vi "UE9 ms Multiple Pulse Output.vi"(8 "error in":errorcluster) -> ()   [LabVIEW 2021]
panel:
  in  "Number of Pulses":u16=1
  in  "Pulse Width (ms)":dbl=10.0 min=1.0 max=260.0 step=1.0
  in  "FirstFound":bool=TRUE
  in  "Address":string="1"
  out "Error Message":string
  # "Demonstrates using a PWM output and a stop timer to create multiple pulses with a pulse width\nfrom 1-260 ms which is variable in 1 ms increments.  Frequency of the pulses is 3.8 Hz.  The PWM\noutput is on FIO0, and the stop timer is on FIO1, so FIO0 must be shorted to FIO1 for the stop\ntimer to work.\n\nThe pulses are negative (signal is normally-high).  If positive pulses are needed, an inverter IC\nshould be put on the signal."
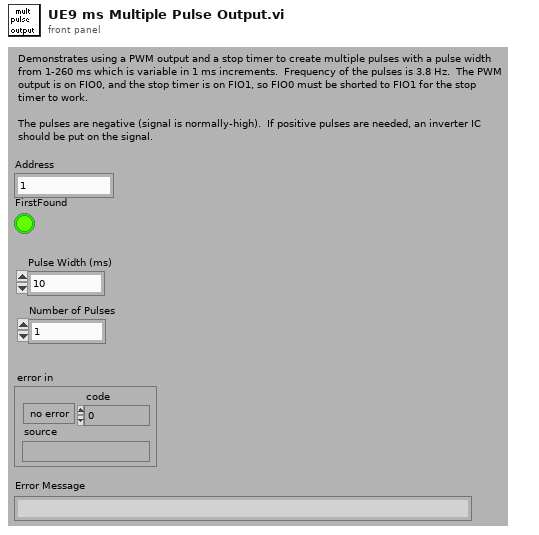
[diagram p1: front panel]
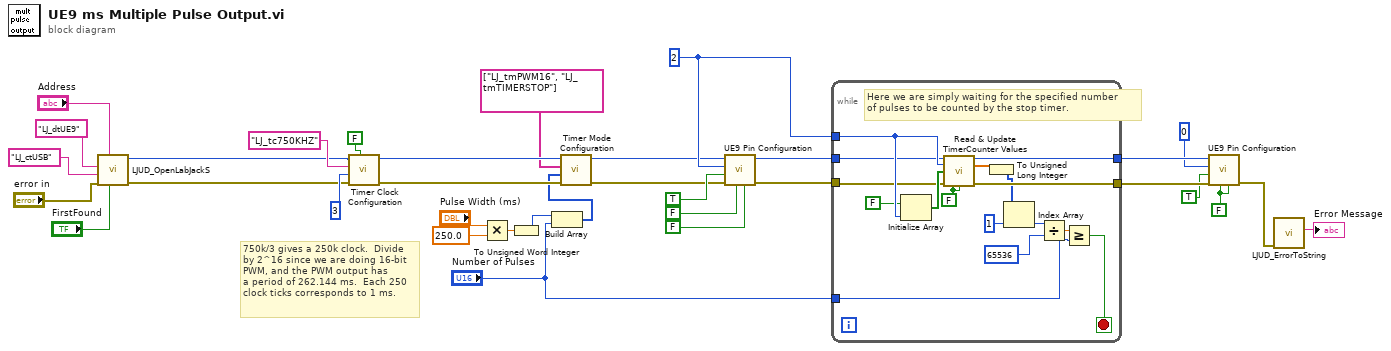
[diagram p0: block diagram]
diagram:
  w8 = FALSE ("Enable Counter0")
  w11 = u8 2 ("Number of Timers Enabled")
  # "750k/3 gives a 250k clock.  Divide\nby 2^16 since we are doing 16-bit\nPWM, and the PWM output has\na period of 262.144 ms.  Each 250\nclock ticks corresponds to 1 ms."
  n1 = call "LJUD_OpenLabJackS.vi"("FirstFound"="FirstFound", "Address"="Address", "error in"="error in", "ConnectionType"="LJ_ctUSB", "DeviceType"="LJ_dtUE9") -> ("error out"=w5:errorcluster, "Handle"=w6:i32)  [unwired: 4 in, 1 out]
  n2 = call "Timer Clock Configuration.vi"("Do Not Do Go()"=FALSE, "error in"=w5, "Timer Clock Divisor"=3, "Timer Clock Base"="LJ_tc750KHZ", "Handle In"=w6) -> ("error out"=w22:errorcluster, "Handle Out"=w21:i32)  [unwired: 5 in]
  n3 = Multiply(x="Pulse Width (ms)", y=250.0) -> (x*y=w15:dbl)
  n4 = To Unsigned Word Integer(number=w15) -> (unsigned 16bit integer=w12:u16)
  n5 = Build Array(w12, "Number of Pulses") -> (w14:u16[])
  n6 = call "Timer Mode Configuration.vi"("error in"=w22, "TimerValues"=w14, "TimerModes"=string[] ["LJ_tmPWM16", "LJ_tmTIMERSTOP"], "Handle In"=w21) -> ("error out"=w3:errorcluster, "Handle Out"=w4:i32)  [unwired: 6 in]
  n7 = call "UE9 Pin Configuration.vi"("Enable Counter1"=FALSE ("Enable Counter0"), "Enable Counter0"=FALSE, "error in"=w3, "Enable DACs"=TRUE ("Enable Counter0"), "Number of Timers Enabled"=w11, "Handle In"=w4) -> ("error out"=w2:errorcluster, "Handle Out"=w1:i32)  [unwired: 4 in]
  n8 = while {
    tunnel: [w50] -> w10
    tunnel: [w48] -> w30
    tunnel: w11 -> [w47]
    tunnel: w1 -> [w45]
    tunnel: w2 -> [w44]
    tunnel: "Number of Pulses" -> [w35]
    stop <- w37 stop-if-true
    w46 = FALSE ("Reset Counter0")
    # "Here we are simply waiting for the specified number\nof pulses to be counted by the stop timer."
    n9 = Initialize Array(FALSE, w47) -> (w49:bool[])
    n10 = call "Read & Update TimerCounter Values.vi"("Handle In"=w45, "# Timers to Read"=w47, "UpdateReset Timers"=w49, "error in"=w44, "Read Counter0"=w46, "Read Counter1"=w46) -> ("Handle Out"=w48:i32, "Timer Value Reads"=w39:dbl[], "error out"=w50:errorcluster)  [unwired: 6 in, 1 out]
    n11 = To Unsigned Long Integer(number=w39) -> (unsigned 32bit integer=w38:u32[])
    n12 = Index Array(array=w38, index=1 ("Index")) -> (element=w40:u32)
    n13 = Divide(x=w40, y=u32 65536) -> (x/y=w41:dbl)
    n14 = Greater Or Equal?(x=w41, y=w35) -> (x >= y?=w37:bool)
  }
  n15 = call "UE9 Pin Configuration.vi"("Enable Counter1"=w8, "Enable Counter0"=w8, "error in"=w10, "Enable DACs"=TRUE, "Number of Timers Enabled"=u8 0 ("# Timers Enabled"), "Handle In"=w30) -> ("error out"=w29:errorcluster)  [unwired: 4 in, 1 out]
  n16 = call "LJUD_ErrorToString.vi"("error in"=w29) -> ("String"=→"Error Message":string)  [unwired: 10 in]
